vi "Write Configuration File.vi"(8 "error in (no error)":errorcluster, 11 "Instrument in":refnum<class "Instrument.lvclass">) -> (0 "error out":errorcluster, 3 "Instrument out":refnum<class "Instrument.lvclass">)   [LabVIEW 2016, in "Instrument.lvclass"]
uses:
  Instrument.lvclass
  Instrument.lvclass/Instrument.ctl
  Configuration/Configuration.lvclass
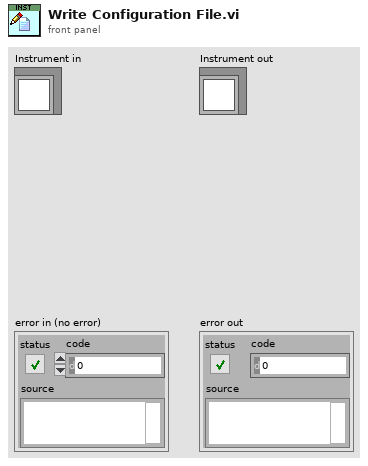
[diagram p1: front panel]
types:
  T1 = typedef "Instrument.lvclass/Configuration--Cluster.ctl" = cluster{"Hardware":T2, "SMO":T3, "DSC":T5}
  T2 = typedef "Instrument.lvclass/HW Configuration--Cluster.ctl" = cluster{"Address":string, "Type":string, "COM Type":string}
  T3 = typedef "Instrument.lvclass/SMO Configuration--Cluster.ctl" = cluster{"Address":string, "Port":u16, "RC Type":T4}
  T4 = typedef "Instrument.lvclass/SMO RC Type--enum.ctl" = enum16{"RC", "STM", "ZMQ"}
  T5 = typedef "Instrument.lvclass/DSC Configuration--Cluster.ctl" = cluster{"Process Name":string}
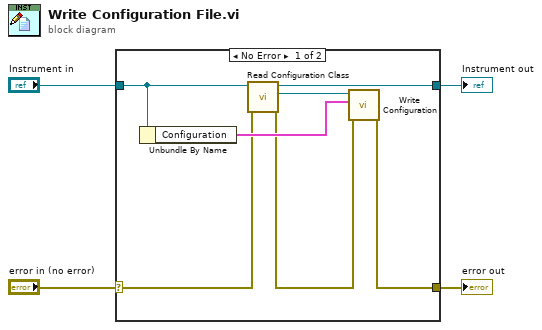
[diagram p0: block diagram]
diagram:
  n1 = case shown="No Error" "error in (no error)" {
    selector: "error in (no error)" -> [w6 w13]
    tunnel: [w11 w12] -> w4
    tunnel: [w9 w13] -> w3
    tunnel: "Instrument in" -> [w7 w12]
    frame No Error {
      n2 = Unbundle By Name(w7) -> ("Configuration"=w8:T1)
      n3 = call "Read Configuration Class.vi"("error in (no error)"=w6, "Instrument in"=w7) -> ("error out"=w5:errorcluster, "Configuration.lvclass"=w10:refnum<class "Configuration.lvclass">, "Instrument out"=w11:refnum<class "Instrument.lvclass">)  [unwired: 7 in]
      n4 = call "Write Configuration.vi"("error in (no error)"=w5, "Variant"=w8, "Configuration in"=w10) -> ("error out"=w9:errorcluster)  [unwired: 7 in, 1 out]
    }
    frame Error {
    }
  }
  "Instrument out" <- w4
  "error out" <- w3
